vi "GF_StringFullTokenizer.vi"(9 "delimiters (\\s,\\t,\\r,\\n)":string[](array[string]), 10 "operators (none)":string[](array[string]), 11 "Input String":string) -> (3 "Token Array":string[](array[string]))   [LabVIEW 2020]
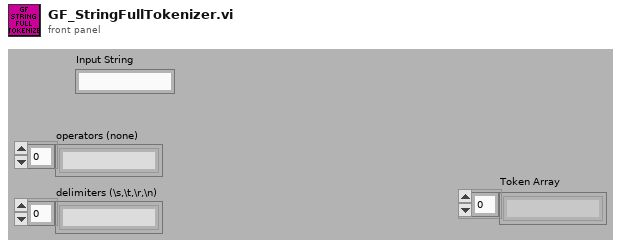
[diagram p1: front panel]
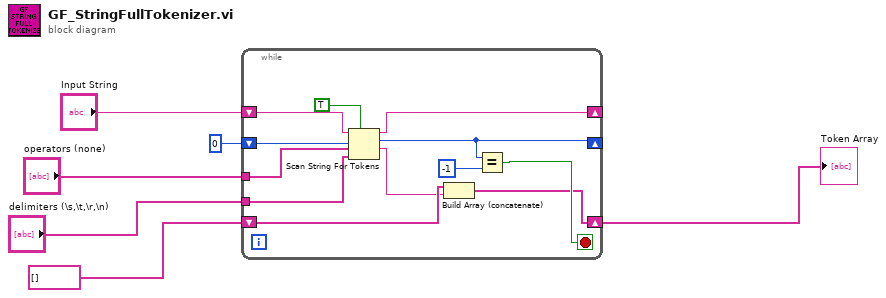
[diagram p0: block diagram]
diagram:
  n1 = while {
    shift-right: [w9] -> _
    shift-left: 0 ("offset") -> [w17]
    shift-right: [w15] -> _
    shift-left: "Input String" -> [w18]
    tunnel: "delimiters (\\s,\\t,\\r,\\n)" -> [w12]
    tunnel: "operators (none)" -> [w11]
    shift-right: [w7] -> w1
    shift-left: string[] [] ("Token Array") -> [w14]
    stop <- w10 stop-if-true
    n2 = Scan String For Tokens(5:TRUE ("allow empty tokens? (F)"), 6:w12, 7:w11, 8:w17, 9:w18) -> (1:w13:string, 2:w9:i32, 3:w15:string)  [unwired: 1 in, 1 out]
    n3 = Build Array (concatenate)(w14, w13) -> (w7:string[])
    n4 = Equal?(x=w9, y=-1 ("offset past token")) -> (x = y?=w10:bool)
  }
  "Token Array" <- w1
